vi "Adjust Dashboard Window.vi"(6 "Sizing Refnums":T1, 9 "Size Constraints":cluster{"min tab width":i32, "w/h":dbl}, 10 "VI":refnum<vi>, 11 "WIn Mode":refnum<notifier>) -> ()   [LabVIEW 2016]
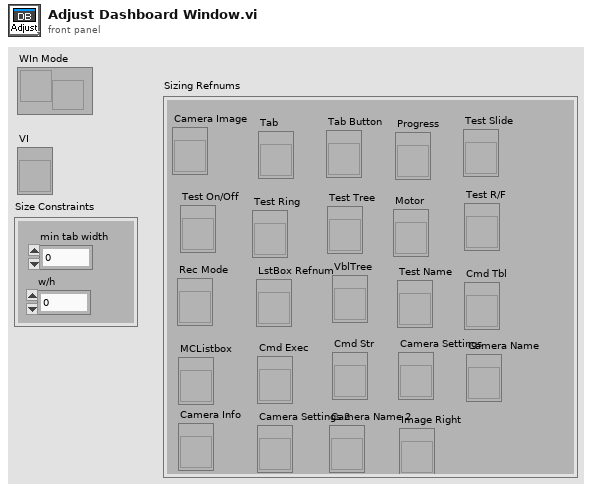
[diagram p1: front panel]
types:
  T1 = cluster{"Camera Image":refnum<vi>, "Tab":refnum<vi>, "Tab Button":refnum<vi>, "Rec Mode":refnum<vi>, "Test Slide":refnum<vi>, "Test On/Off":refnum<vi>, "Test Ring":refnum<vi>, "Test R/F":refnum<vi>, "Test Name":refnum<vi>, "Motor":refnum<vi>, "Progress":refnum<vi>, "LstBox Refnum":refnum<vi>, "Test Tree":refnum<vi>, "VblTree":refnum<vi>, "Cmd Tbl":refnum<vi>, "MCListbox":refnum<vi>, "Cmd Exec":refnum<vi>, "Cmd Str":refnum<vi>, "Camera Settings":refnum<vi>, "Camera Name":refnum<vi>, "Camera Info":refnum<vi>, "Camera Settings 2":refnum<vi>, "Camera Name 2":refnum<vi>, "Image Right":refnum<vi>}
  T2 = typedef "LVPointTypeDef.ctl" = cluster{"Horizontal":i16, "Vertical":i16}
  T3 = typedef "LVRectTypeDef.ctl" = cluster{"Left":i16, "Top":i16, "Right":i16, "Bottom":i16}
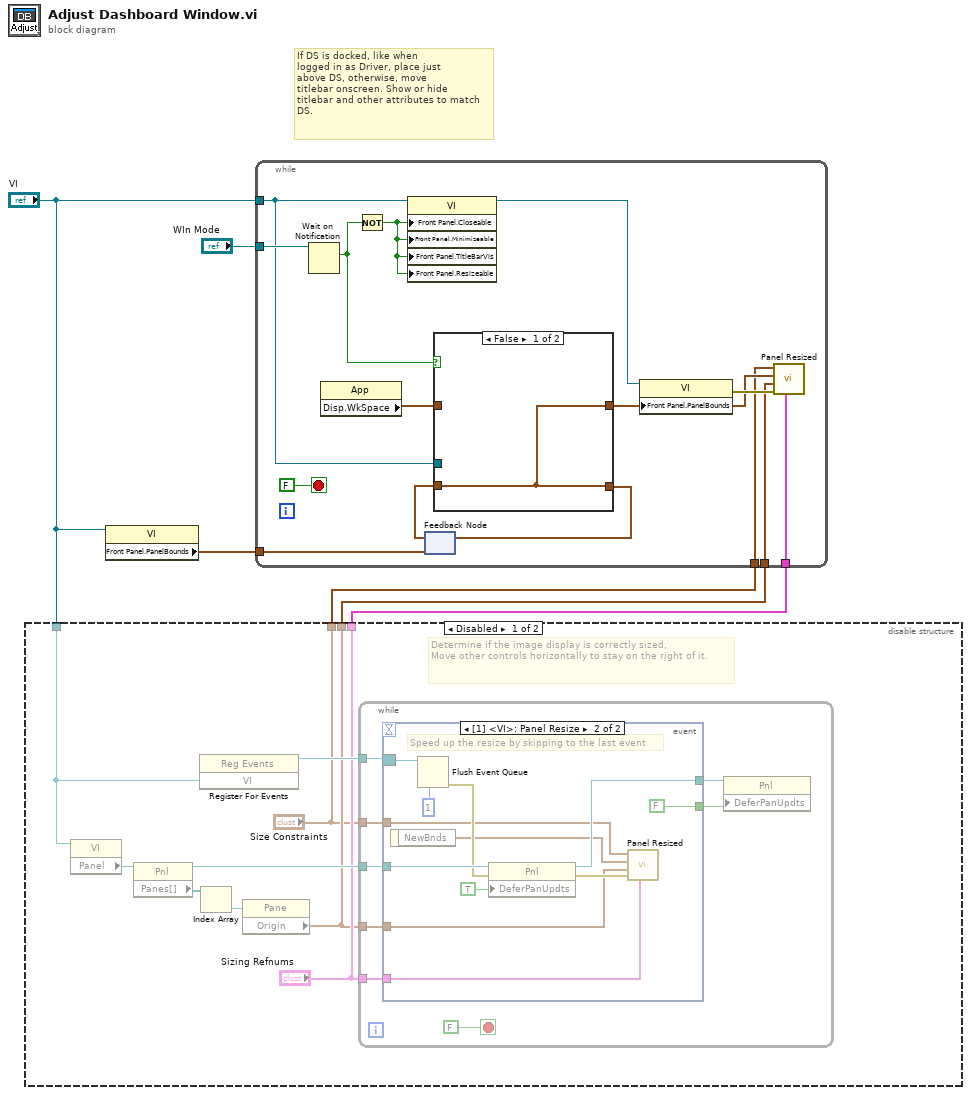
[diagram p0: block diagram]
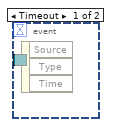
[diagram p2: hidden frame]
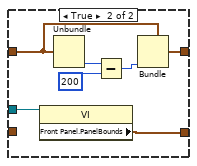
[diagram p4: hidden frame]
diagram:
  # "If DS is docked, like when\nlogged in as Driver, place just\nabove DS, otherwise, move\ntitlebar onscreen. Show or hide\ntitlebar and other attributes to match\nDS."
  n1 = disable-structure shown="Disabled" {
    disable-tunnel: ["Sizing Refnums" _] -> w5
    disable-tunnel: [w9 _] -> w4
    disable-tunnel: ["Size Constraints" _] -> w3
    disable-tunnel: "VI" -> [w7 _]
    frame Disabled {
      # "Determine if the image display is correctly sized,\nMove other controls horizontally to stay on the right of it."
      n2 = property class="VI"(reference=w7) -> ("Panel"=w14:refnum<vi>)  [unwired: 1 in, 2 out]
      n3 = property class="Pnl"(reference=w14) -> (reference out=w11:refnum<vi>, "Panes[]"=w13:refnum<vi>[])  [unwired: 1 in, 1 out]
      n4 = register-events(w7) -> (reference out=w15:refnum<event-registration>)  [unwired: 2 in, 1 out]
      n5 = Index Array(array=w13) -> (element=w12:refnum<vi>)  [unwired: 1 in]
      n6 = property class="Pane"(reference=w12) -> ("Origin"=w9:T2)  [unwired: 1 in, 2 out]
      n7 = while {
        tunnel: w15 -> [w22]
        tunnel: "Sizing Refnums" -> [w21]
        tunnel: "Size Constraints" -> [w20]
        tunnel: w9 -> [w19]
        tunnel: w11 -> [w18]
        stop <- FALSE stop-if-true
        n8 = event shown="[1] <VI>: Panel Resize" {
          selector: w22 -> [_ w32]
          dyn-events: _ -> [_ _]
          timeout: _ -> [_ _]
          tunnel: w21 -> [_ w24]
          tunnel: w20 -> [_ w27]
          tunnel: w19 -> [_ w25]
          tunnel: w18 -> [_ w35]
          tunnel: [_ FALSE ("Defer Panel Updates")] -> w17
          tunnel: [_ w29] -> w16
          event Timeout {
            n9 = event-data() -> ()  [unwired: 1 in, 3 out]
          }
          event Panel Resize {
            # "Speed up the resize by skipping to the last event"
            n10 = event-data() -> ("NewBnds"=w26:T3)  [unwired: 1 in]
            n11 = Flush Event Queue(0:w32, 5:1 ("keep most recent")) -> (11:w30:errorcluster)  [unwired: 4 in, 2 out]
            n12 = property class="Pnl"(reference=w35, error in=w30, "DeferPanUpdts"=TRUE ("Defer Panel Updates")) -> (reference out=w29:refnum<vi>, error out=w28:errorcluster)
            n13 = call "Panel Resized.vi"("Sizing Refnums"=w24, "error in (no error)"=w28, "Origin"=w25, "NewBnds"=w26, "Size Constraints"=w27) -> ()  [unwired: 6 in, 1 out]
          }
        }
        n14 = property class="Pnl"(reference=w16, "DeferPanUpdts"=w17) -> ()  [unwired: 1 in, 2 out]
      }
    }
    frame Enabled {
    }
  }
  n15 = property class="VI"(reference="VI") -> ("Front Panel.PanelBounds"=w2:T3)  [unwired: 1 in, 2 out]
  n16 = while {
    tunnel: "WIn Mode" -> [w49]
    tunnel: "VI" -> [w40]
    tunnel: w5 -> [w45]
    tunnel: w4 -> [w44]
    tunnel: w3 -> [w42]
    tunnel: w2 -> [w37]
    stop <- FALSE stop-if-true
    n17 = Wait on Notification(notifier=w49) -> (notification=w41:bool)  [unwired: 3 in, 3 out]
    n18 = property class="App"() -> ("Disp.WkSpace"=w48:T3)  [unwired: 2 in, 2 out]
    n19 = Not(x=w41) -> (.not. x?=w36:bool)
    n20 = property class="VI"(reference=w40, "Front Panel.Closeable"=w36, "Front Panel.Minimizeable"=w36, "Front Panel.TitleBarVis"=w36, "Front Panel.Resizeable"=w36) -> (reference out=w47:refnum<vi>)  [unwired: 1 in, 1 out]
    n21 = feedback #1(w37) -> (w38:T3)
    n22 = case shown="False" w41 {
      tunnel: w48 -> [_ w54]
      tunnel: [w51 w55] -> w43
      tunnel: w40 -> [_ w53]
      tunnel: [w51 w52] -> w39
      tunnel: w38 -> [w51 _]
      frame False {
      }
      frame True {
        n23 = property class="VI"(reference=w53) -> ("Front Panel.PanelBounds"=w52:T3)  [unwired: 1 in, 2 out]
        n24 = Unbundle(w54) -> ("Bottom"=w58:i16)  [unwired: 3 out]
        n25 = Subtract(x=w58, y=200) -> (x-y=w56:i32)
        n26 = Bundle(cluster=w54, "Bottom"=w56) -> (w55:T3)  [unwired: 3 out]
      }
    }
    n27 = feedback-in #1(w39) -> ()
    n28 = property class="VI"(reference=w47, "Front Panel.PanelBounds"=w43) -> (error out=w46:errorcluster)  [unwired: 1 in, 1 out]
    n29 = call "Panel Resized.vi"("Sizing Refnums"=w45, "error in (no error)"=w46, "Origin"=w44, "NewBnds"=w43, "Size Constraints"=w42) -> ()  [unwired: 6 in, 1 out]
  }
